vi "InitMH_AnyThread.vi"(8 "error in (no error)":errorcluster, 9 "Mode":T2 items=["HIST"=0, "T2"=2, "T3"=3], 10 "refsource":T1, 11 "Library Version":string="1.0") -> (0 "error out":errorcluster, 2 "Init Info":T3, 3 "DevIdx":i32)   [LabVIEW 2019]
uses:
  MH_InitInfo.ctl
  MH_MeasMode.ctl
  MH_RefSource.ctl
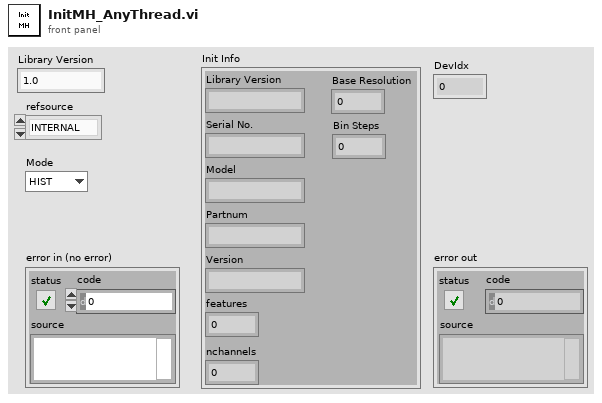
[diagram p1: front panel]
types:
  T1 = typedef "MH_RefSource.ctl" = enum16{"INTERNAL", "EXTERNAL_10MHZ", "WR_MASTER_GENERIC", "WR_SLAVE_GENERIC", "WR_GRANDM_GENERIC", "EXTN_GPS_PPS", "EXTN_GPS_PPS_UART", "WR_MASTER_MHARP", "WR_SLAVE_MHARP", "WR_GRANDM_MHARP"}
  T2 = typedef "MH_MeasMode.ctl" = i32
  T3 = typedef "MH_InitInfo.ctl" = cluster{"Library Version":string, "Serial No.":string, "Model":string, "Partnum":string, "Version":string, "features":i32, "nchannels":i32, "Base Resolution":dbl, "Bin Steps":i32}
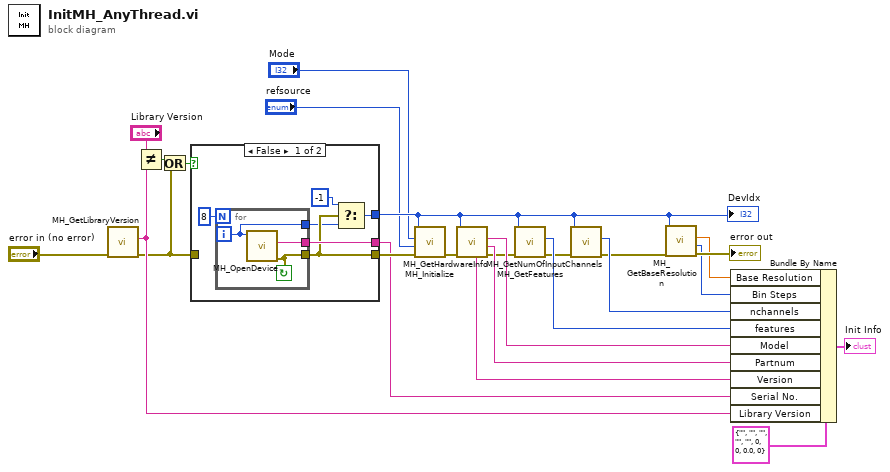
[diagram p0: block diagram]
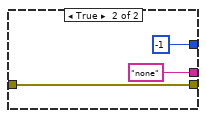
[diagram p2: hidden frame]
diagram:
  n1 = call "MH_GetLibraryVersion.vi"("error in (no error)"="error in (no error)") -> ("error out"=w6:errorcluster, "Version"=w14:string)  [unwired: 8 in, 1 out]
  n2 = Not Equal?(x="Library Version", y=w14) -> (x != y?=w24:bool)
  n3 = Or(x=w24, y=w6) -> (x .or. y?=w23:bool)
  n4 = case shown="False" w23 {
    tunnel: [w27 -1 ("return type")] -> w5
    tunnel: [w30 "none" ("serial")] -> w16
    tunnel: [w29 w35] -> w22
    tunnel: w6 -> [_ w35]
    frame False {
      n5 = for {
        N: 8 -> [_]
        tunnel: [w33] -> w29
        tunnel: [w32] -> w30
        tunnel: [w34] -> w28
        i -> [w34]
        stop <- w33 continue-if-true
        n6 = call "MH_OpenDevice.vi"("devidx"=w34) -> ("error out"=w33:errorcluster, "serial"=w32:string)  [unwired: 8 in, 1 out]
      }
      n7 = Select(t=-1, s=w29, f=w28) -> (s? t:f=w27:i32)
    }
    frame True {
    }
  }
  "DevIdx" <- w5
  n8 = call "MH_Initialize.vi"("error in (no error)"=w22, "refsource"="refsource", "mode"="Mode", "devidx"=w5) -> ("error out"=w21:errorcluster)  [unwired: 6 in, 1 out]
  n9 = call "MH_GetHardwareInfo.vi"("error in (no error)"=w21, "devidx"=w5) -> ("error out"=w12:errorcluster, "Partnum"=w19:string, "Model"=w20:string, "Version"=w18:string)  [unwired: 5 in, 1 out]
  n10 = call "MH_GetFeatures.vi"("error in (no error)"=w12, "devidx"=w5) -> ("error out"=w4:errorcluster, "features"=w17:i32)  [unwired: 7 in, 1 out]
  n11 = call "MH_GetNumOfInputChannels.vi"("error in (no error)"=w4, "devidx"=w5) -> ("error out"=w1:errorcluster, "nchannels"=w11:i32)  [unwired: 7 in, 1 out]
  n12 = call "MH_GetBaseResolution.vi"("error in (no error)"=w1, "devidx"=w5) -> ("error out"=→"error out":errorcluster, "binsteps"=w9:i32, "resolution"=w8:dbl)  [unwired: 6 in, 1 out]
  n13 = Bundle By Name(cluster=T3 {"Library Version"="", "Serial No."="", "Model"="", "Partnum"="", "Version"="", "features"=0, "nchannels"=0, "Base Resolution"=0.0, "Bin Steps"=0} ("Init"), "Base Resolution"=w8, "Bin Steps"=w9, "nchannels"=w11, "features"=w17, "Model"=w20, "Partnum"=w19, "Version"=w18, "Serial No."=w16, "Library Version"=w14) -> (→"Init Info":T3)
